vi "Create Arbitrary Waveform.vi"(8 "error in (no error)":errorcluster, 9 "Arbitrary Waveform Data":dbl[](array[numeric]), 10 "Arbitrary Waveform Name":string, 11 "VISA resource name":refnum<visa-resource-name>) -> (0 "error out":errorcluster, 3 "VISA resource name out":refnum<visa-resource-name>)   [LabVIEW 2015, in "Fluke 28x Series.lvlib"]
doc: "Creates and saves an arbitrary (user-defined) waveform in non-volatile memory.\n\n<B>Note</B>: Call the Configure Arbitrary Waveform VI to set the arbitrary waveform as the active function."
uses:
  <instrlib>/Fluke 28x Series/Fluke 28x Series.lvlib
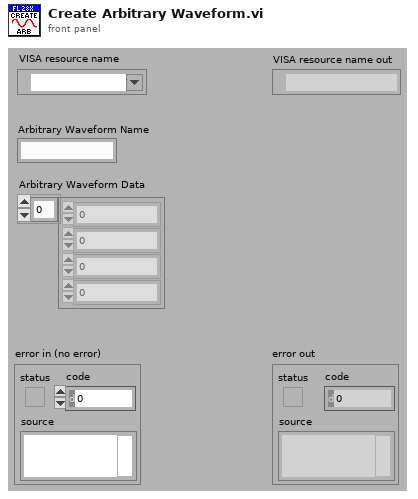
[diagram p1: front panel]
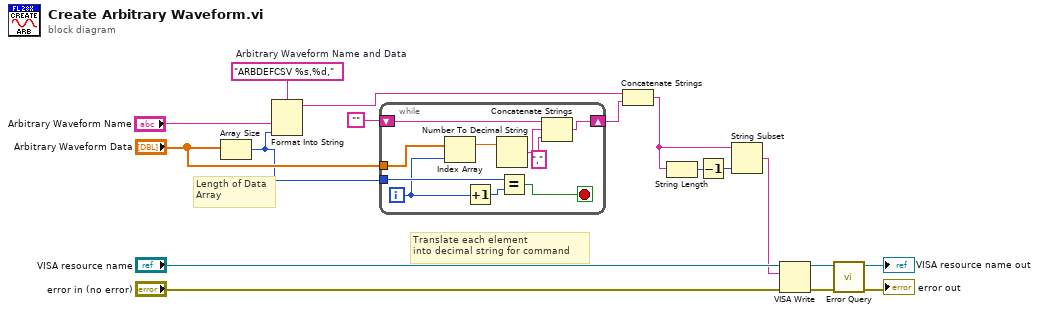
[diagram p0: block diagram]
diagram:
  w11 = "ARBDEFCSV %s,%d,"  # Arbitrary Waveform Name and Data
  # "Translate each element\ninto decimal string for command"
  # "Length of Data\nArray"
  n1 = Array Size(array="Arbitrary Waveform Data") -> (size(s)=w8:i32)
  n2 = Format Into String(format string=w11, "Arbitrary Waveform Name", w8) -> (resulting string=w7:string)  [unwired: 2 in, 1 out]
  n3 = while {
    shift-right: [w23] -> w6
    shift-left: "" -> [w21]
    tunnel: "Arbitrary Waveform Data" -> [w27]
    tunnel: w8 -> [w25]
    i -> [w18]
    stop <- w24 stop-if-true
    n4 = Index Array(array=w27, index=w18) -> (element=w19:dbl)
    n5 = Increment(x=w18) -> (x+1=w26:i32)
    n6 = Number To Decimal String(number=w19) -> (decimal integer string=w22:string)  [unwired: 1 in]
    n7 = Equal?(x=w25, y=w26) -> (x = y?=w24:bool)
    n8 = Concatenate Strings(w21, w22, "," ("string")) -> (w23:string)
  }
  n9 = Concatenate Strings(w7, w6) -> (w4:string)
  n10 = String Length(string=w4) -> (length=w2:i32)
  n11 = Decrement(x=w2) -> (x-1=w1:i32)
  n12 = String Subset(string=w4, length (rest)=w1) -> (substring=w3:string)  [unwired: 1 in]
  n13 = VISA Write(VISA resource name="VISA resource name", write buffer=w3, error in (no error)="error in (no error)") -> (VISA resource name out=w15:refnum<visa-resource-name>, error out=w14:errorcluster)  [unwired: 1 out]
  n14 = call <instrlib>:"Error Query.vi"("error in (no error)"=w14, "VISA resource name"=w15) -> ("error out"=→"error out":errorcluster, "VISA resource name out"=→"VISA resource name out":refnum<visa-resource-name>)  [unwired: 6 in, 2 out]
